vi "ButtonPress.vi"(11 "Button In":bool) -> (3 "Button Pressed?":bool)   [LabVIEW 2017]
doc: "When using the Joystick Get Values function, pushing a joystick button will cause the button to read TRUE until the button is released. This means that you will most likely read multiple TRUE values for each press. Use this vi to create only one TRUE value each time the button is pressed."
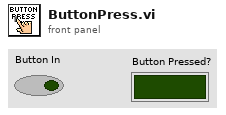
[diagram p1: front panel]
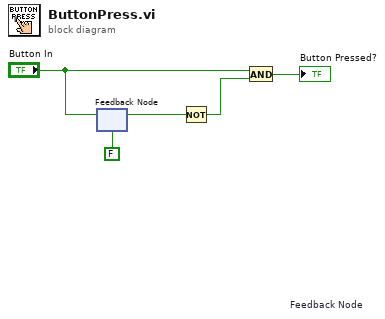
[diagram p0: block diagram]
diagram:
  n1 = feedback #1 "Feedback Node"(FALSE ("Button In")) -> (w5:bool)
  n2 = feedback-in #1("Button In") -> ()
  n3 = Not(x=w5) -> (.not. x?=w4:bool)
  n4 = And(x="Button In", y=w4) -> (x .and. y?=→"Button Pressed?":bool)
